vi "UsrProfiles-Source-Internal user prof name.vi"() -> (3 "Previous session profile name":string)   [LabVIEW 2020]
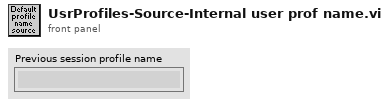
[diagram p1: front panel]
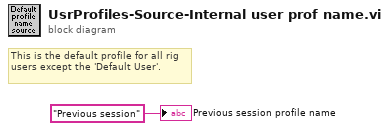
[diagram p0: block diagram]
diagram:
  # "This is the default profile for all rig users except the 'Default User'."
  "Previous session profile name" <- "Previous session" ("element")
